vi "Set Numeric Text.vi"(7 "Treatment of Infinity/NaN":T1, 8 "error in (no error)":errorcluster, 10 "Numeric Text":string, 11 "JSON Scalar in":refnum<class "JSON Scalar.lvclass">) -> (0 "error out":errorcluster, 3 "JSON Scalar out":refnum<class "JSON Scalar.lvclass">)   [LabVIEW 2020, in "Library Commun.lvlib" / "JSON Scalar.lvclass"]
uses:
  JSON Scalar.lvclass
  Infinity&NaN.ctl
  JSON Scalar.lvclass/JSON Scalar.ctl
  Quote and Escape JSON string.vi
  support/JSON support.lvlib
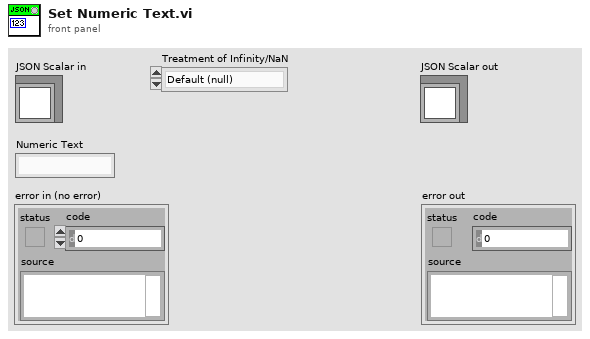
[diagram p1: front panel]
types:
  T1 = typedef "Library Commun.lvlib/JSON support.lvlib/Infinity&NaN.ctl" = enum16{"Default (null)", "Extended", "LabVIEW extensions"}
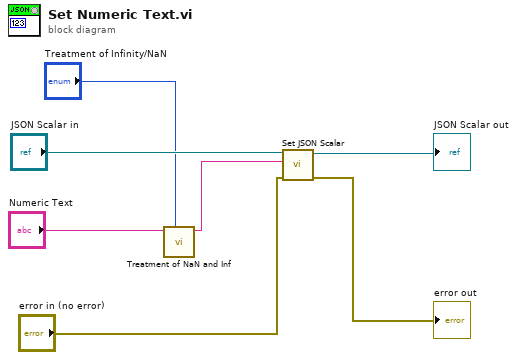
[diagram p0: block diagram]
diagram:
  n1 = call "Treatment of NaN and Inf.vi"("Treatment of Infinity/NaN"="Treatment of Infinity/NaN", "Numeric Text"="Numeric Text") -> ("<JSON>"=w3:string)  [unwired: 9 in]
  n2 = call "Set JSON Scalar.vi"("error in (no error)"="error in (no error)", "LabVIEW Text"=w3, "JSON Scalar in"="JSON Scalar in") -> ("error out"=→"error out":errorcluster, "JSON Scalar out"=→"JSON Scalar out":refnum<class "JSON Scalar.lvclass">)  [unwired: 7 in]
